vi "Boiler.vi"() -> ()   [LabVIEW 2020]
doc: "This VI simulates the operation of a boiler. There is a proper sequence of steps that must be followed in order to start it up:\n\n1) Run Interlock Closed\n2) Boiler Reset\n3) Start Sequence\n4) Wait for 10 second Pre-Purge to complete\n5) Pilot\n6) Flame Sensor Value over 30%\n7) Forced Draft Fan on\n8) Fuel Control Valve Position between 10% and 75% open\n\nOnce the boiler is running it can be shut down by any of the following:\n1) Shutdown button\n2) Run Interlock Open\n3) Forced Draft Fan Off\n4) Fuel Control Valve Position Less than 10% or greater than 75% open\n\nShutdown is followed by a 10 second Purge before the system resumes the initial state."
uses:
  Controls/Boiler States Enum.ctl
  Controls/File Command Enum.ctl
  Controls/Timer Commands Enum.ctl
panel:
  in  "App Stop":bool
  in  "Boiler Simulation Controls":T1 {"Flame Sensor Value (%)" scale=0.0..100.0}
  in  "Boiler Controls":T2 {"Fuel Control Valve Position (% Open)" scale=0.0..100.0}
  out "Boiler Status Indicators":T3 {"Time Count (s)" format="%.2f"}
  # "On"
  # "Off"
  # "Closed"
  # "Open"
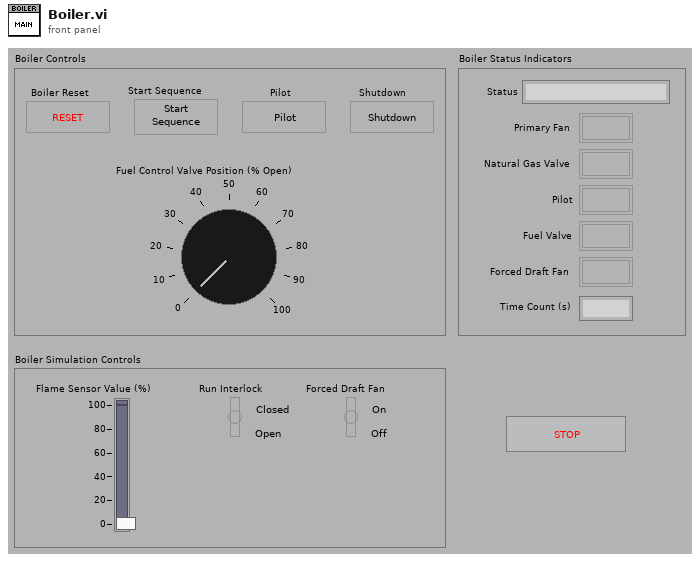
[diagram p1: front panel]
types:
  T1 = cluster{"Flame Sensor Value (%)":dbl, "Run Interlock":bool, "Forced Draft Fan":bool}
  T2 = cluster{"Shutdown":bool, "Pilot Button":bool, "Start Sequence":bool, "Boiler Reset":bool, "Fuel Control Valve Position (% Open)":dbl}
  T3 = cluster{"Time Count (s)":dbl, "Status":string, "Forced Draft Fan":bool, "Fuel Valve":bool, "Pilot Indicator":bool, "Natural Gas Valve":bool, "Primary Fan":bool}
  T4 = typedef "File Command Enum.ctl" = enum16{"Open File", "Write Log Data", "Close File"}
  T5 = cluster{"Time Count (s)":dbl, "Status":string, "Forced Draft Fan":bool, "Fuel Valve":bool, "Pilot":bool, "Natural Gas Valve":bool, "Primary Fan":bool}
  T6 = typedef "Boiler States Enum.ctl" = enum16{"Reset Values", "Lockout", "Ready", "Pre-Purge", "Pre-Purge Complete", "Pilot On", "Boiler Ready", "Boiler Running", "Purge"}
  T7 = typedef "Timer Commands Enum.ctl" = enum16{"Start Timer", "Check Timer"}
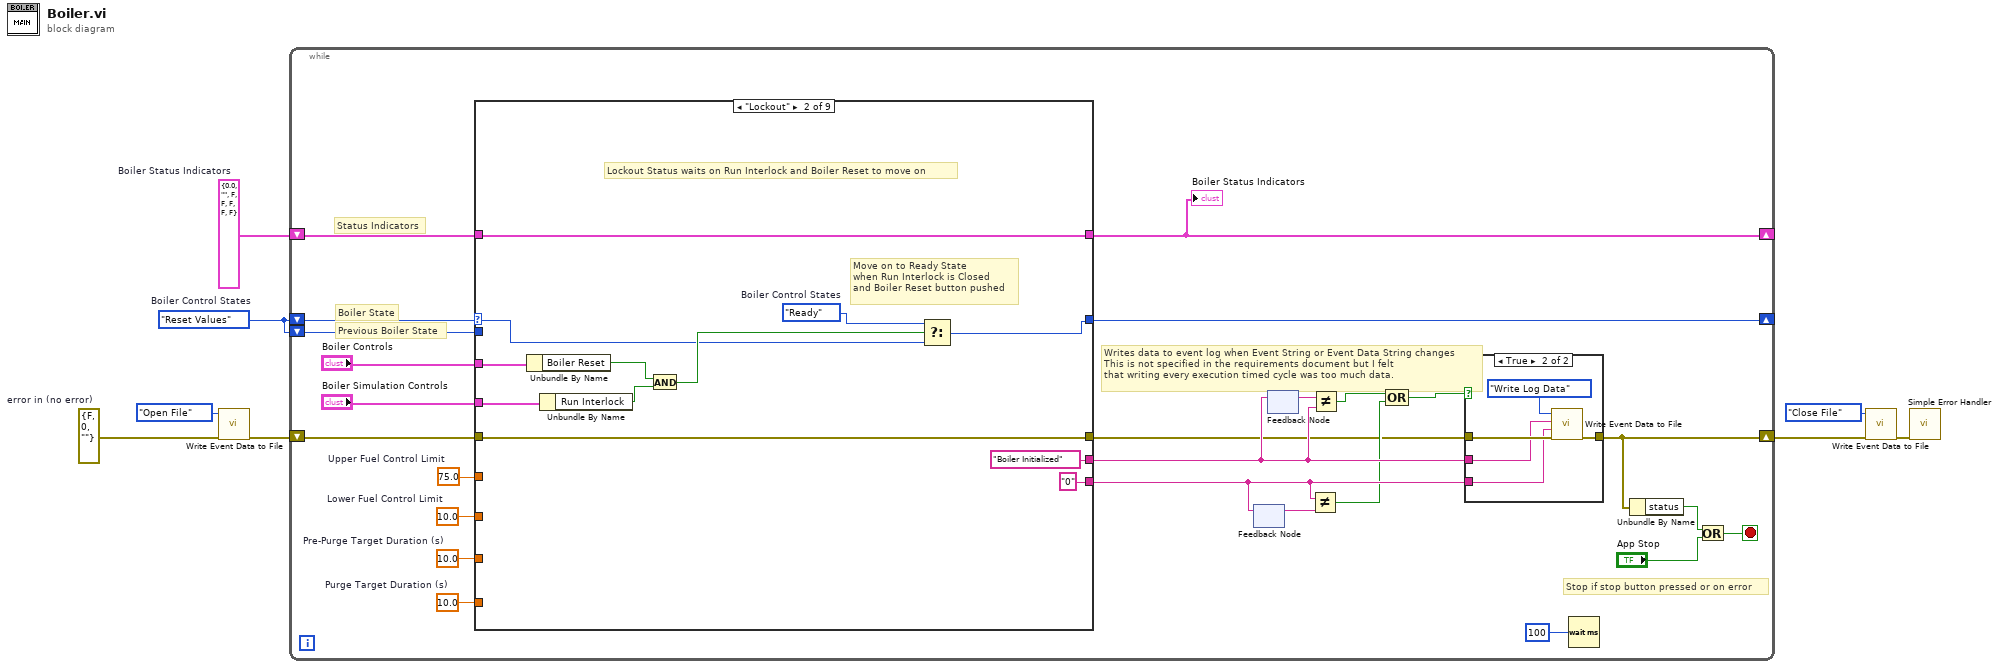
[diagram p0: block diagram]
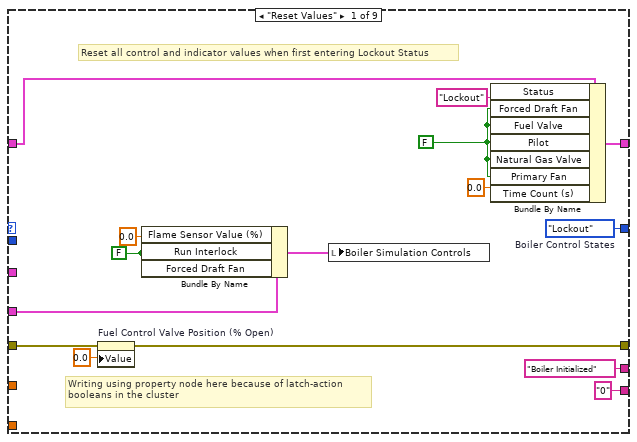
[diagram p3: hidden frame]
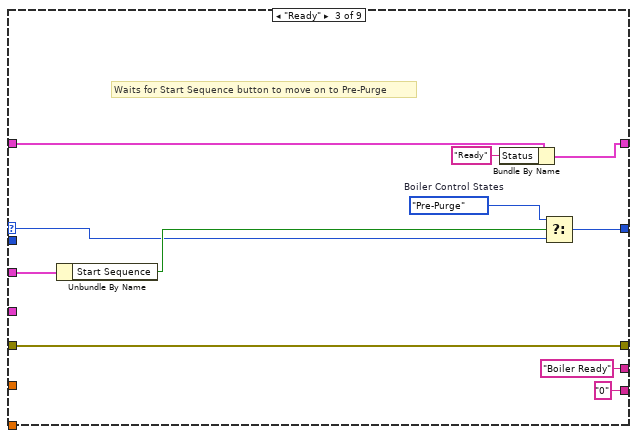
[diagram p4: hidden frame]
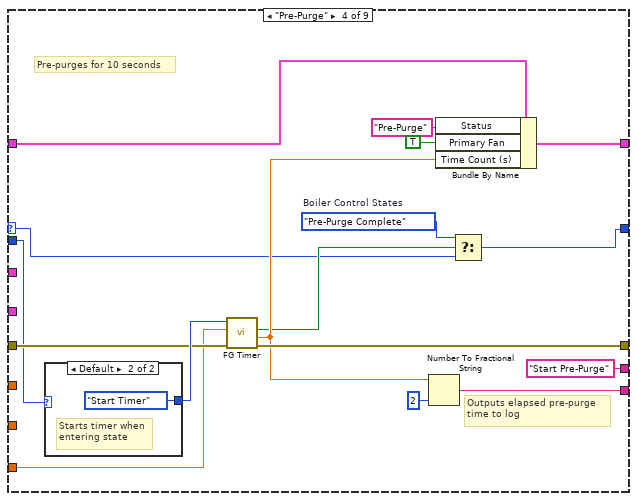
[diagram p5: hidden frame]
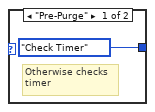
[diagram p6: hidden frame]
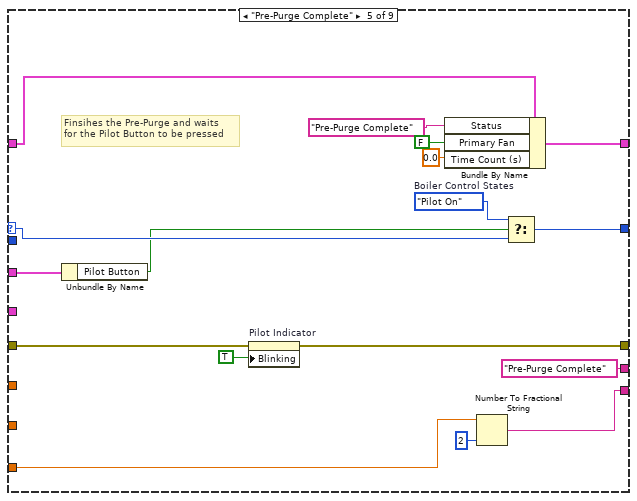
[diagram p7: hidden frame]
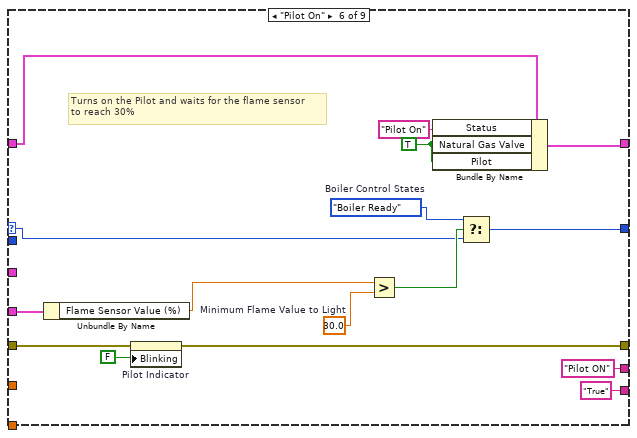
[diagram p8: hidden frame]
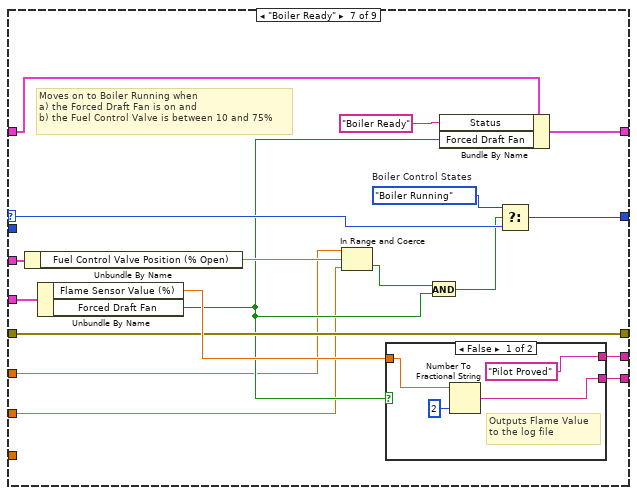
[diagram p9: hidden frame]
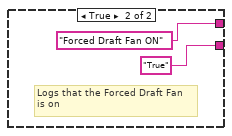
[diagram p10: hidden frame]
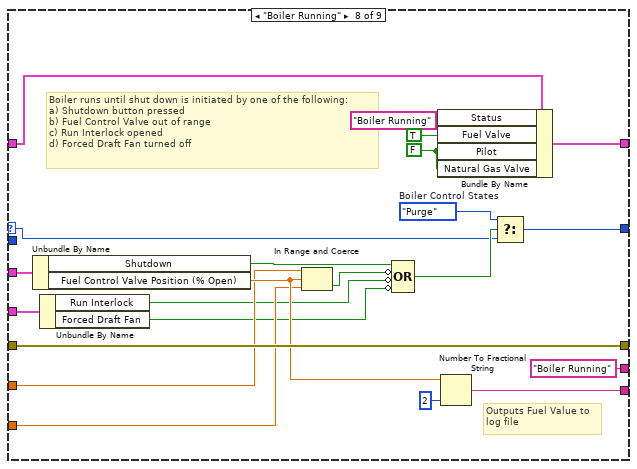
[diagram p11: hidden frame]
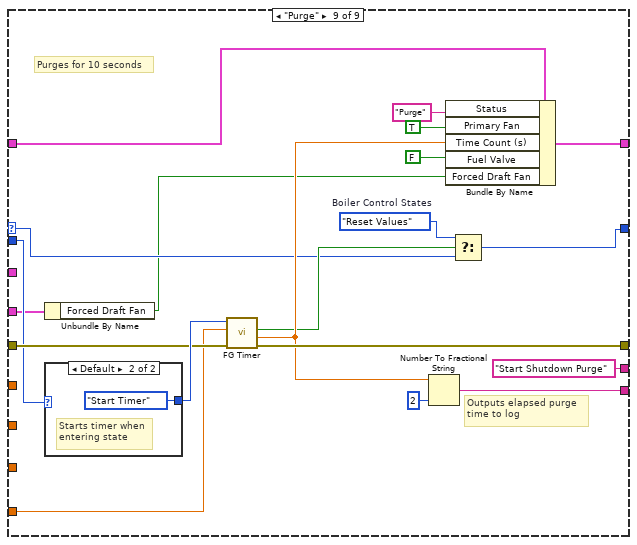
[diagram p12: hidden frame]
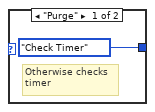
[diagram p13: hidden frame]
diagram:
  w3 = errorcluster {"status"=FALSE, "code"=0, "source"=""}  # error in (no error)
  w8 = T5 {"Time Count (s)"=0.0, "Status"="", "Forced Draft Fan"=FALSE, "Fuel Valve"=FALSE, "Pilot"=FALSE, "Natural Gas Valve"=FALSE, "Primary Fan"=FALSE}  # Boiler Status Indicators
  w1 = Boiler_States_Enum."Reset Values"  # Boiler Control States
  n1 = call "Write Event Data to File.vi"("error in (no error)"=w3, "File Operations"=File_Command_Enum."Open File") -> ("error out"=w4:errorcluster)  [unwired: 9 in]
  n2 = while {
    shift-right: [w23] -> _
    shift-left: w1 -> [w33]
    shift-right: [w29] -> _
    shift-left: w8 -> [w30]
    shift-right: [w22] -> w7
    shift-left: w4 -> [w27]
    shift-left: w1 -> [w17]
    stop <- w24 stop-if-true
    w18 = 10.0  # Purge Target Duration (s)
    w20 = 75.0  # Upper Fuel Control Limit
    w19 = 10.0  # Lower Fuel Control Limit
    w21 = 10.0  # Pre-Purge Target Duration (s)
    # "Previous Boiler State"
    # "Writes data to event log when Event String or Event Data String changes\nThis is not specified in the requirements document but I felt\nthat writing every execution timed cycle was too much data."
    # "Stop if stop button pressed or on error"
    # "Status Indicators"
    # "Boiler State"
    n3 = case shown="\"Lockout\"" w33 {
      selector: w33 -> [_ w55 w67 w79 w101 w116 w142 w155 w179]
      tunnel: "Boiler Controls" -> [_ w59 w70 _ w98 _ w137 w170 _]
      tunnel: "Boiler Simulation Controls" -> [w48 w66 _ _ _ w120 w141 w165 w177]
      tunnel: w30 -> [w50 w63 w77 w88 w113 w129 w147 w175 w189]
      tunnel: [w51 w63 w76 w87 w112 w121 w145 w174 w188] -> w29
      tunnel: w27 -> [w41 w62 w72 w93 w104 w126 w138 w166 w194]
      tunnel: [w40 w62 w72 w89 w103 w124 w138 w166 w190] -> w9
      tunnel: [w49 w65 w71 w83 w100 w115 w143 w157 w184] -> w23
      tunnel: ["Boiler Initialized" "Boiler Initialized" "Boiler Ready" "Start Pre-Purge" "Pre-Purge Complete" "Pilot ON" w146 "Boiler Running" "Start Shutdown Purge"] -> w15
      tunnel: ["0" "0" "0" w91 w107 "True" w140 w168 w192] -> w12
      tunnel: w21 -> [_ _ _ w80 w106 _ _ _ _]
      tunnel: w20 -> [_ _ _ _ _ _ w131 w162 _]
      tunnel: w19 -> [_ _ _ _ _ _ w130 w163 _]
      tunnel: w18 -> [_ _ _ _ _ _ _ _ w181]
      tunnel: w17 -> [_ _ _ w78 _ _ _ _ w178]
      frame "Reset Values" {
        w45 = FALSE ("Run Interlock")
        w49 = Boiler_States_Enum."Lockout"  # Boiler Control States
        w52 = FALSE
        # "Writing using property node here because of latch-action\nbooleans in the cluster"
        # "Reset all control and indicator values when first entering Lockout Status"
        n4 = property on="Fuel Control Valve Position (% Open)" class="Knob (strict)"(error in=w41, "Value"=0.0) -> (error out=w40:errorcluster)  [unwired: 1 in, 1 out]
        n5 = Bundle By Name(cluster=w48, "Flame Sensor Value (%)"=0.0, "Run Interlock"=w45, "Forced Draft Fan"=w45) -> (w47:T1)
        n6 = local write "Boiler Simulation Controls"(w47) -> ()
        n7 = Bundle By Name(cluster=w50, "Status"="Lockout", "Forced Draft Fan"=w52, "Fuel Valve"=w52, "Pilot"=w52, "Natural Gas Valve"=w52, "Primary Fan"=w52, "Time Count (s)"=0.0) -> (w51:T5)
      }
      frame "Lockout" {
        w64 = Boiler_States_Enum."Ready"  # Boiler Control States
        # "Lockout Status waits on Run Interlock and Boiler Reset to move on"
        # "Move on to Ready State\nwhen Run Interlock is Closed\nand Boiler Reset button pushed"
        n8 = Unbundle By Name(w59) -> ("Boiler Reset"=w58:bool)
        n9 = Unbundle By Name(w66) -> ("Run Interlock"=w57:bool)
        n10 = And(x=w58, y=w57) -> (x .and. y?=w56:bool)
        n11 = Select(t=w64, s=w56, f=w55) -> (s? t:f=w65:T6)
      }
      frame "Ready" {
        w68 = Boiler_States_Enum."Pre-Purge"  # Boiler Control States
        # "Waits for Start Sequence button to move on to Pre-Purge"
        n12 = Unbundle By Name(w70) -> ("Start Sequence"=w69:bool)
        n13 = Bundle By Name(cluster=w77, "Status"="Ready") -> (w76:T5)
        n14 = Select(t=w68, s=w69, f=w67) -> (s? t:f=w71:T6)
      }
      frame "Pre-Purge" {
        w81 = Boiler_States_Enum."Pre-Purge Complete"  # Boiler Control States
        # "Pre-purges for 10 seconds"
        # "Outputs elapsed pre-purge\ntime to log"
        n15 = case shown="Default" w78 {
          tunnel: [Timer_Commands_Enum."Check Timer" ("Timer Commands") Timer_Commands_Enum."Start Timer" ("Timer Commands")] -> w94
          frame "Pre-Purge" {
            # "Otherwise checks\ntimer"
          }
          frame Default {
            # "Starts timer when\nentering state"
          }
        }
        n16 = call "FG Timer.vi"("error in (no error)"=w93, "Target Duration (s)"=w80, "Timer Commands"=w94) -> ("error out"=w89:errorcluster, "Elapsed Time"=w86:dbl, "Done?"=w82:bool)  [unwired: 6 in]
        n17 = Number To Fractional String(number=w86, precision (6)=i16 2) -> (F-format string=w91:string)  [unwired: 2 in]
        n18 = Bundle By Name(cluster=w88, "Status"="Pre-Purge", "Primary Fan"=TRUE, "Time Count (s)"=w86) -> (w87:T5)
        n19 = Select(t=w81, s=w82, f=w79) -> (s? t:f=w83:T6)
      }
      frame "Pre-Purge Complete" {
        w99 = Boiler_States_Enum."Pilot On"  # Boiler Control States
        # "Finsihes the Pre-Purge and waits\nfor the Pilot Button to be pressed"
        n20 = Unbundle By Name(w98) -> ("Pilot Button"=w97:bool)
        n21 = property on="Pilot Indicator" class="Bool (strict)"(error in=w104, "Blinking"=TRUE) -> (error out=w103:errorcluster)  [unwired: 1 in, 1 out]
        n22 = Bundle By Name(cluster=w113, "Status"="Pre-Purge Complete", "Primary Fan"=FALSE, "Time Count (s)"=0.0) -> (w112:T5)
        n23 = Number To Fractional String(number=w106, precision (6)=i16 2) -> (F-format string=w107:string)  [unwired: 2 in]
        n24 = Select(t=w99, s=w97, f=w101) -> (s? t:f=w100:T6)
      }
      frame "Pilot On" {
        w114 = Boiler_States_Enum."Boiler Ready"  # Boiler Control States
        w118 = 30.0  # Minimum Flame Value to Light
        w127 = TRUE ("Natural Gas Valve")
        # "Turns on the Pilot and waits for the flame sensor\nto reach 30%"
        n25 = Unbundle By Name(w120) -> ("Flame Sensor Value (%)"=w119:dbl)
        n26 = property on="Pilot Indicator" class="Bool (strict)"(error in=w126, "Blinking"=FALSE) -> (error out=w124:errorcluster)  [unwired: 1 in, 1 out]
        n27 = Greater?(x=w119, y=w118) -> (0:w117:bool)
        n28 = Bundle By Name(cluster=w129, "Status"="Pilot On", "Natural Gas Valve"=w127, "Pilot"=w127) -> (w121:T5)
        n29 = Select(t=w114, s=w117, f=w116) -> (s? t:f=w115:T6)
      }
      frame "Boiler Ready" {
        w132 = Boiler_States_Enum."Boiler Running"  # Boiler Control States
        # "Moves on to Boiler Running when\na) the Forced Draft Fan is on and\nb) the Fuel Control Valve is between 10 and 75%"
        n30 = Unbundle By Name(w137) -> ("Fuel Control Valve Position (% Open)"=w136:dbl)
        n31 = Unbundle By Name(w141) -> ("Flame Sensor Value (%)"=w139:dbl, "Forced Draft Fan"=w134:bool)
        n32 = In Range and Coerce(upper limit=w131, x=w136, lower limit=w130) -> (In Range?=w135:bool)  [unwired: 1 out]
        n33 = case shown="False" w134 {
          tunnel: ["Pilot Proved" "Forced Draft Fan ON"] -> w146
          tunnel: [w150 "True"] -> w140
          tunnel: w139 -> [w149 _]
          frame False {
            # "Outputs Flame Value\nto the log file"
            n34 = Number To Fractional String(number=w149, precision (6)=i16 2) -> (F-format string=w150:string)  [unwired: 2 in]
          }
          frame True {
            # "Logs that the Forced Draft Fan\nis on"
          }
        }
        n35 = And(x=w135, y=w134) -> (x .and. y?=w133:bool)
        n36 = Bundle By Name(cluster=w147, "Status"="Boiler Ready", "Forced Draft Fan"=w134) -> (w145:T5)
        n37 = Select(t=w132, s=w133, f=w142) -> (s? t:f=w143:T6)
      }
      frame "Boiler Running" {
        w154 = Boiler_States_Enum."Purge"  # Boiler Control States
        w171 = FALSE ("Pilot")
        # "Boiler runs until shut down is initiated by one of the following:\na) Shutdown button pressed\nb) Fuel Control Valve out of range\nc) Run Interlock opened\nd) Forced Draft Fan turned off"
        # "Outputs Fuel Value to\nlog file"
        n38 = Unbundle By Name(w170) -> ("Shutdown"=w161:bool, "Fuel Control Valve Position (% Open)"=w164:dbl)
        n39 = Unbundle By Name(w165) -> ("Run Interlock"=w159:bool, "Forced Draft Fan"=w158:bool)
        n40 = In Range and Coerce(upper limit=w162, x=w164, lower limit=w163) -> (In Range?=w160:bool)  [unwired: 1 out]
        n41 = Compound Arithmetic op=OR(w161, invert w160, invert w159, invert w158) -> (w156:bool)
        n42 = Bundle By Name(cluster=w175, "Status"="Boiler Running", "Fuel Valve"=TRUE, "Pilot"=w171, "Natural Gas Valve"=w171) -> (w174:T5)
        n43 = Number To Fractional String(number=w164, precision (6)=i16 2) -> (F-format string=w168:string)  [unwired: 2 in]
        n44 = Select(t=w154, s=w156, f=w155) -> (s? t:f=w157:T6)
      }
      frame "Purge" {
        w182 = Boiler_States_Enum."Reset Values"  # Boiler Control States
        # "Purges for 10 seconds"
        # "Outputs elapsed purge\ntime to log"
        n45 = Unbundle By Name(w177) -> ("Forced Draft Fan"=w176:bool)
        n46 = case shown="Default" w178 {
          tunnel: [Timer_Commands_Enum."Check Timer" ("Timer Commands") Timer_Commands_Enum."Start Timer" ("Timer Commands")] -> w195
          frame "Purge" {
            # "Otherwise checks\ntimer"
          }
          frame Default {
            # "Starts timer when\nentering state"
          }
        }
        n47 = call "FG Timer.vi"("error in (no error)"=w194, "Target Duration (s)"=w181, "Timer Commands"=w195) -> ("error out"=w190:errorcluster, "Elapsed Time"=w187:dbl, "Done?"=w183:bool)  [unwired: 6 in]
        n48 = Number To Fractional String(number=w187, precision (6)=i16 2) -> (F-format string=w192:string)  [unwired: 2 in]
        n49 = Bundle By Name(cluster=w189, "Status"="Purge", "Primary Fan"=TRUE, "Time Count (s)"=w187, "Fuel Valve"=FALSE, "Forced Draft Fan"=w176) -> (w188:T5)
        n50 = Select(t=w182, s=w183, f=w179) -> (s? t:f=w184:T6)
      }
    }
    "Boiler Status Indicators" <- w29
    n51 = feedback-in #1(w12) -> ()
    n52 = feedback #1() -> (w13:string)  [unwired: 1 in]
    n53 = feedback-in #2(w15) -> ()
    n54 = feedback #2() -> (w16:string)  [unwired: 1 in]
    n55 = Not Equal?(x=w12, y=w13) -> (x != y?=w11:bool)
    n56 = Not Equal?(x=w16, y=w15) -> (x != y?=w14:bool)
    n57 = Compound Arithmetic op=OR(w14, w11) -> (w10:bool)
    n58 = case shown="True" w10 {
      tunnel: w9 -> [w34 w39]
      tunnel: [w34 w38] -> w22
      tunnel: w15 -> [_ w37]
      tunnel: w12 -> [_ w36]
      frame False {
      }
      frame True {
        n59 = call "Write Event Data to File.vi"("error in (no error)"=w39, "Event Data String"=w36, "Event String"=w37, "File Operations"=File_Command_Enum."Write Log Data") -> ("error out"=w38:errorcluster)  [unwired: 7 in]
      }
    }
    n60 = Wait (ms)(milliseconds to wait=u32 100) -> ()  [unwired: 1 out]
    n61 = Unbundle By Name(w22) -> ("status"=w26:bool)
    n62 = Or(x=w26, y="App Stop") -> (x .or. y?=w24:bool)
  }
  n63 = call "Write Event Data to File.vi"("error in (no error)"=w7, "File Operations"=File_Command_Enum."Close File") -> ("error out"=w6:errorcluster)  [unwired: 9 in]
  n64 = call <vilib>:"Simple Error Handler.vi"("error in (no error)"=w6) -> ()  [unwired: 4 in, 5 out]
